vi "myRIO_Gil_RT__randomizeMinMax__v2.vi"(9 "Input_Increment":u16=1 min=1 step=1, 10 "Input_Min":u16=1 min=1 step=1, 11 "Input_Max":u16=1 min=1 step=1) -> (3 "Output":u16)   [LabVIEW 2014]
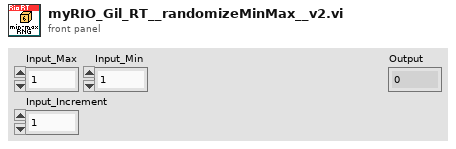
[diagram p1: front panel]
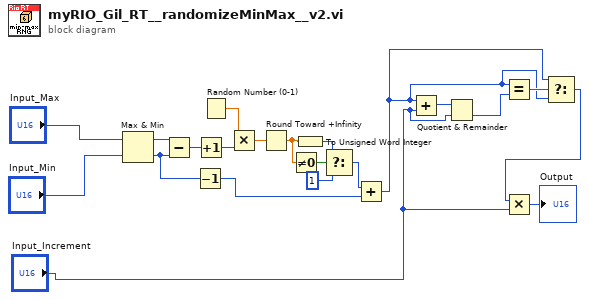
[diagram p0: block diagram]
diagram:
  n1 = Max & Min(x="Input_Max", y="Input_Min") -> (max(x,y)=w21:u16, min(x,y)=w17:u16)
  n2 = Subtract(x=w21, y=w17) -> (x-y=w20:u16)
  n3 = Decrement(x=w17) -> (x-1=w12:u16)
  n4 = Increment(x=w20) -> (x+1=w19:u16)
  n5 = Random Number (0-1)() -> (number: 0 to 1=w18:dbl)
  n6 = Multiply(x=w18, y=w19) -> (x*y=w16:dbl)
  n7 = Round Toward +Infinity(x=w16) -> (ceil(x): smallest int >= x=w7:dbl)
  n8 = Not Equal To 0?(x=w7) -> (x != 0?=w15:bool)
  n9 = To Unsigned Word Integer(number=w7) -> (unsigned 16bit integer=w8:u16)
  n10 = Select(t=w8, s=w15, f=u16 1) -> (s? t:f=w13:u16)
  n11 = Add(x=w13, y=w12) -> (x+y=w2:u16)
  n12 = Add(x=w2, y="Input_Increment") -> (x+y=w6:u16)
  n13 = Quotient & Remainder(x=w6, y="Input_Increment") -> (floor(x/y)=w4:u16)  [unwired: 1 out]
  n14 = Equal?(x=w2, y=w4) -> (x = y?=w3:bool)
  n15 = Select(t=w2, s=w3, f=w2) -> (s? t:f=w1:u16)
  n16 = Multiply(x=w1, y="Input_Increment") -> (x*y=→"Output":u16)
